vi "Write Roles.vi"(8 "error in (no error)":errorcluster, 10 "Roles":T1, 11 "PreparePenaltyAllyPlay in":refnum<class "PreparePenaltyAllyPlay.lvclass">) -> (0 "error out":errorcluster, 3 "PreparePenaltyAllyPlay out":refnum<class "PreparePenaltyAllyPlay.lvclass">)   [LabVIEW 2023, in "PreparePenaltyAllyPlay.lvclass"]
uses:
  PreparePenaltyAllyPlay.lvclass
  AttackerAimGoalRole_class/AttackerAimGoalRole.lvclass
  PenaltyDefenseRole_class/PenaltyDefenseRole.lvclass
  PreparePenaltyAllyPlay.lvclass/PreparePenaltyAllyPlay.ctl
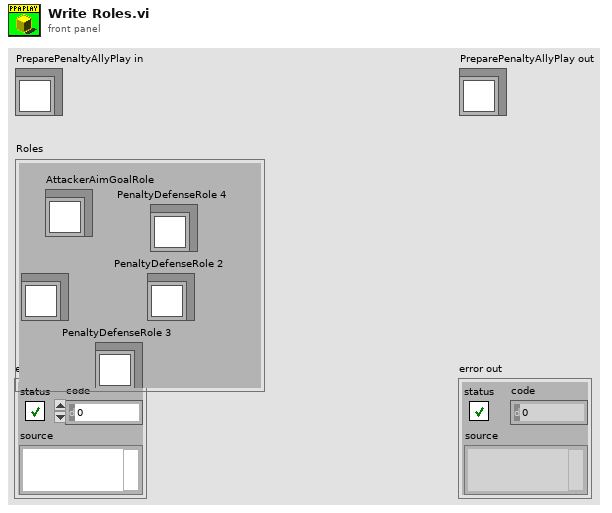
[diagram p1: front panel]
types:
  T1 = cluster{"AttackerAimGoalRole":refnum<class "AttackerAimGoalRole.lvclass">, "PenaltyDefenseRole 4":refnum<class "PenaltyDefenseRole.lvclass">, "PenaltyDefenseRole 1":refnum<class "PenaltyDefenseRole.lvclass">, "PenaltyDefenseRole 2":refnum<class "PenaltyDefenseRole.lvclass">, "PenaltyDefenseRole 3":refnum<class "PenaltyDefenseRole.lvclass">}
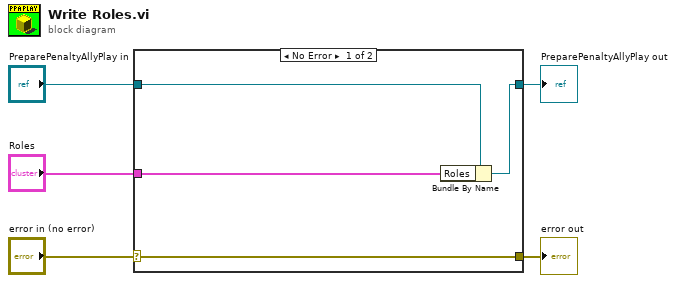
[diagram p0: block diagram]
diagram:
  n1 = case shown="No Error" "error in (no error)" {
    selector: "error in (no error)" -> [w9 w10]
    tunnel: [w9 w10] -> w4
    tunnel: [w7 w11] -> w2
    tunnel: "PreparePenaltyAllyPlay in" -> [w8 w11]
    tunnel: "Roles" -> [w6 _]
    frame No Error {
      n2 = Bundle By Name(cluster=w8, "Roles"=w6) -> (w7:refnum<class "PreparePenaltyAllyPlay.lvclass">)
    }
    frame Error {
    }
  }
  "error out" <- w4
  "PreparePenaltyAllyPlay out" <- w2
